vi "Generate File Path.vi"(8 "error in (no error)":errorcluster) -> (0 "error out":errorcluster, 3 "file path":path)   [LabVIEW 2021]
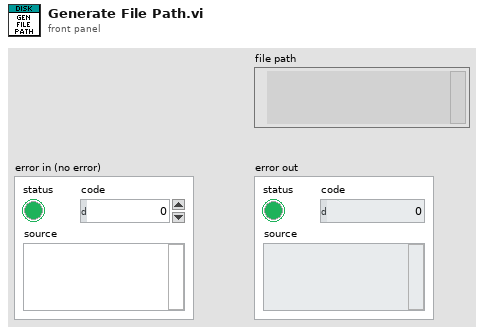
[diagram p1: front panel]
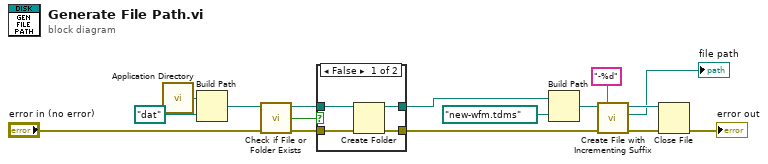
[diagram p0: block diagram]
diagram:
  n1 = call <vilib>:"Application Directory.vi"() -> ("Application Directory"=w16:path)
  n2 = Build Path(base path=w16, name or relative path=path "dat") -> (appended path=w13:path)
  n3 = call <vilib>:"Check if File or Folder Exists.vi"("error in (no error)"="error in (no error)", "path"=w13) -> ("error out"=w12:errorcluster, "file or folder exists?"=w10:bool, "dup path"=w11:path)  [unwired: 7 in]
  n4 = case shown="False" w10 {
    tunnel: w12 -> [w20 w22]
    tunnel: [w19 w22] -> w6
    tunnel: w11 -> [w18 w21]
    tunnel: [w17 w21] -> w9
    frame False {
      n5 = Create Folder(path (use dialog)=w18, error in=w20) -> (created path=w17:path, error out=w19:errorcluster)  [unwired: 1 in, 1 out]
    }
    frame True {
    }
  }
  n6 = Build Path(base path=w9, name or relative path=path "new-wfm.tdms") -> (appended path=w7:path)
  n7 = call <vilib>:"Create File with Incrementing Suffix.vi"("format string (\" (%d)\")"="-%d" ("format string (\" (%d)\")"), "error in (no error)"=w6, "file path"=w7) -> ("error out"=w4:errorcluster, "actual path"=→"file path":path, "refnum out"=w3:refnum<file>)  [unwired: 6 in]
  n8 = Close File(refnum=w3, error in=w4) -> (error out=→"error out":errorcluster)  [unwired: 1 out]
